vi "Write Type.vi"(8 "error in (no error)":errorcluster, 10 "Type":T1[](array[typedef]) items=["J", "K", "T", "E", "R", "S", "N", "B"], 11 "9213 in":refnum<class "9213.lvclass">) -> (0 "error out":errorcluster, 3 "9213 out":refnum<class "9213.lvclass">)   [LabVIEW 2019, in "Modules.lvlib" / "9213.lvclass"]
uses:
  9213.lvclass
  Thermocouple Type.ctl
  9213.lvclass/9213.ctl
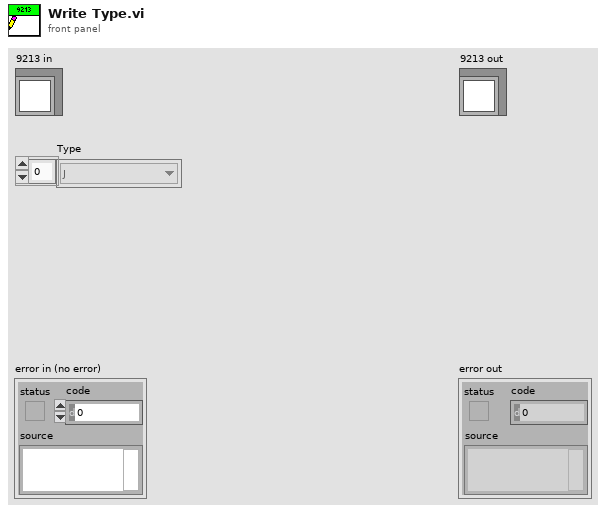
[diagram p1: front panel]
types:
  T1 = typedef "Modules.lvlib/9213.lvclass/Thermocouple Type.ctl" = u8
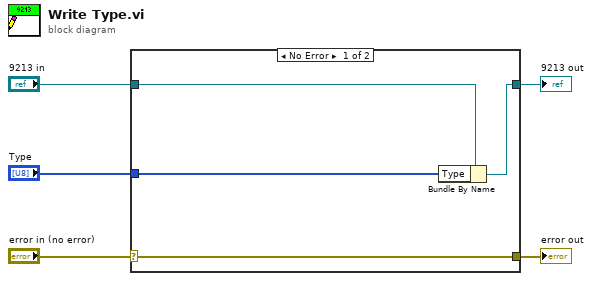
[diagram p0: block diagram]
diagram:
  n1 = case shown="No Error" "error in (no error)" {
    selector: "error in (no error)" -> [w9 w10]
    tunnel: [w9 w10] -> w4
    tunnel: [w7 w11] -> w2
    tunnel: "9213 in" -> [w8 w11]
    tunnel: "Type" -> [w6 _]
    frame No Error {
      n2 = Bundle By Name(cluster=w8, "Type"=w6) -> (w7:refnum<class "9213.lvclass">)
    }
    frame Error {
    }
  }
  "error out" <- w4
  "9213 out" <- w2
